vi "Read DSC-Traces.vi"(8 "Error In":errorcluster, 11 "KIT-QA in":refnum<class "KIT-QA.lvclass">) -> (0 "Error Out":errorcluster, 3 "KIT-QA out":refnum<class "KIT-QA.lvclass">)   [LabVIEW 2016, in "KIT-QA.lvlib" / "KIT-QA.lvclass"]
doc: "Read some traces from DSC database."
uses:
  KIT-QA.lvclass
  KIT-QA.lvclass/KIT-QA.ctl
  <vilib>/Waveform/WDTOps.llb/WDT Waveform Duration DBL.vi
  <vilib>/lvdsc/historical/Read Traces (Numeric).vi
  <vilib>/lvdsc/NI_DSC.lvlib
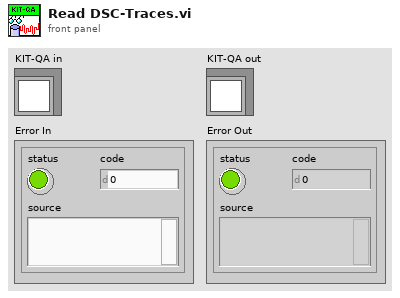
[diagram p1: front panel]
types:
  T1 = cluster{"interpolate data (F)":bool, "extrapolate to now (F)":bool, "remove data breaks (F)":bool, "interpolation interval (1 s)":dbl, "maintain trending info (T)":bool}
  T2 = cluster{"timestamps":timestamp[], "data":dbl[]}[]
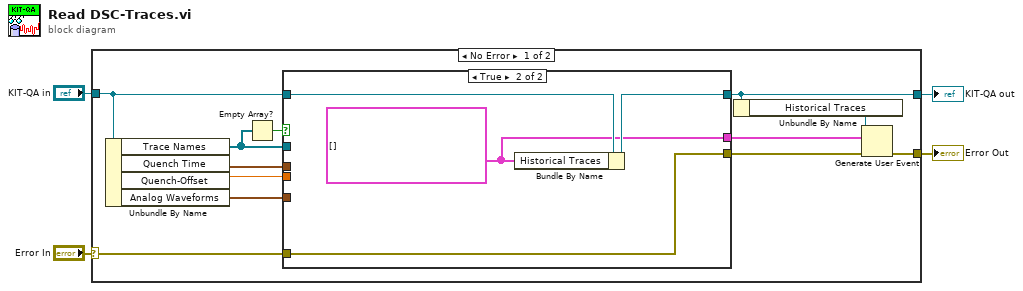
[diagram p0: block diagram]
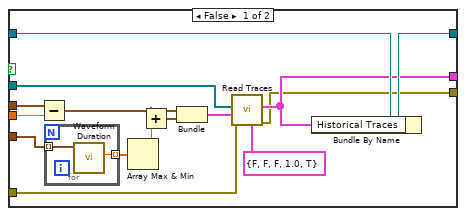
[diagram p2: hidden frame]
diagram:
  n1 = case shown="No Error" "Error In" {
    selector: "Error In" -> [w16 w39]
    tunnel: [w9 w39] -> w3
    tunnel: [w6 w38] -> w1
    tunnel: "KIT-QA in" -> [w12 w38]
    frame No Error {
      n2 = Unbundle By Name(w12) -> ("Trace Names"=w7:refnum<k21>[], "Quench Time"=w15:timestamp, "Quench-Offset"=w14:dbl[unit], "Analog Waveforms"=w13:waveform(dbl)[])
      n3 = Empty Array?(array=w7) -> (empty?=w8:bool)
      n4 = case shown="True" w8 {
        tunnel: w7 -> [w31 _]
        tunnel: w16 -> [w30 w34]
        tunnel: w15 -> [w18 _]
        tunnel: w14 -> [w29 _]
        tunnel: w13 -> [w27 _]
        tunnel: w12 -> [w22 w37]
        tunnel: [w21 w36] -> w6
        tunnel: [w20 w35] -> w11
        tunnel: [w19 w34] -> w10
        frame False {
          n5 = Subtract(x=w18, y=w29) -> (x-y=w26:timestamp)
          n6 = for {
            tunnel: w27 -> [w33] mode=indexing
            tunnel: [w32] -> w25 mode=indexing
            n7 = call-poly <vilib>:"Waveform Duration.vi"("waveform in"=w33) -> ("duration"=w32:dbl)  [unwired: 8 in, 2 out]
          }
          n8 = Array Max & Min(array=w25) -> (max value=w17:dbl)  [unwired: 3 out]
          n9 = Add(x=w26, y=w17) -> (x+y=w24:timestamp)
          n10 = Bundle(w26, w24) -> (w28:cluster{timestamp, timestamp})  [unwired: 1 in]
          n11 = call-poly <vilib>:"Read Traces.vi"("options"=T1 {"interpolate data (F)"=FALSE, "extrapolate to now (F)"=FALSE, "remove data breaks (F)"=FALSE, "interpolation interval (1 s)"=1.0, "maintain trending info (T)"=TRUE}, "error in (no error)"=w30, "time interval"=w28, "trace names"=w31) -> ("error out"=w19:errorcluster, "historical traces"=w20:T2)  [unwired: 4 in, 2 out]
          n12 = Bundle By Name(cluster=w22, "Historical Traces"=w20) -> (w21:refnum<class "KIT-QA.lvclass">)
        }
        frame True {
          w35 = T2 [] ("Historical Traces")
          n13 = Bundle By Name(cluster=w37, "Historical Traces"=w35) -> (w36:refnum<class "KIT-QA.lvclass">)
        }
      }
      n14 = Unbundle By Name(w6) -> ("Historical Traces"=w5:refnum<user-event>)
      n15 = Generate User Event(user event=w5, event data cluster=w11, error in=w10) -> (error out=w9:errorcluster)  [unwired: 1 in, 1 out]
    }
    frame Error {
    }
  }
  "Error Out" <- w3
  "KIT-QA out" <- w1
